vi "_PC_Pub_CreateFilePath.vi"(8 "error in (no error)":errorcluster, 9 "ExtName":string="tdms", 10 "FileName":string="Spectra", 11 "FolderName":string="MSData") -> (0 "error out":errorcluster, 3 "appended path":path)   [LabVIEW 2018]
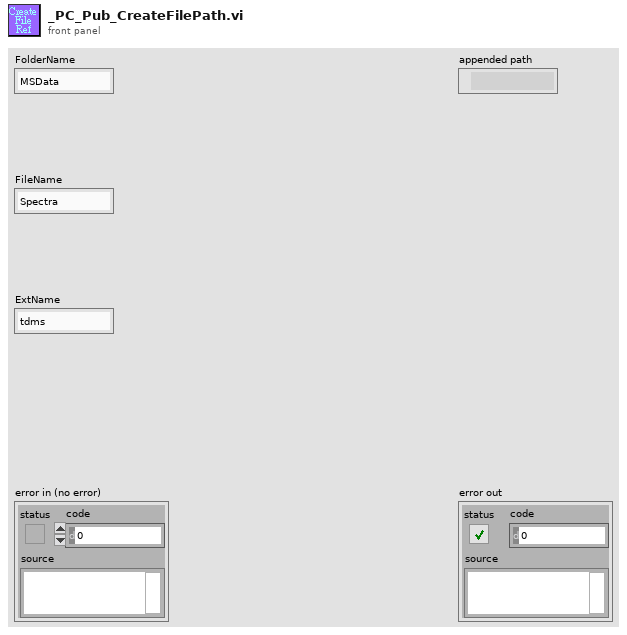
[diagram p1: front panel]
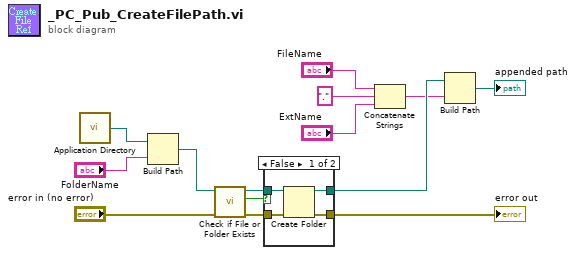
[diagram p0: block diagram]
diagram:
  n1 = call <vilib>:"Application Directory.vi"() -> ("Application Directory"=w14:path)
  n2 = Build Path(base path=w14, name or relative path="FolderName") -> (appended path=w9:path)
  n3 = call <vilib>:"Check if File or Folder Exists.vi"("error in (no error)"="error in (no error)", "path"=w9) -> ("error out"=w10:errorcluster, "file or folder exists?"=w12:bool, "dup path"=w11:path)  [unwired: 7 in]
  n4 = case shown="False" w12 {
    tunnel: w11 -> [w18 w20]
    tunnel: w10 -> [w17 w19]
    tunnel: [w16 w19] -> w6
    tunnel: [w15 w20] -> w8
    frame False {
      n5 = Create Folder(path (use dialog)=w18, error in=w17) -> (created path=w15:path, error out=w16:errorcluster)  [unwired: 1 in, 1 out]
    }
    frame True {
    }
  }
  "error out" <- w6
  n6 = Concatenate Strings("FileName", ".", "ExtName") -> (w1:string)
  n7 = Build Path(base path=w8, name or relative path=w1) -> (appended path=→"appended path":path)
